vi "Snell_law.vi"(10 "Refr index":dbl=7.5, 11 "Angle in ext (deg)":dbl=7.5) -> (2 "Angle out int (deg)":dbl=7.5, 3 "Angle out int (rad)":dbl=7.5)   [LabVIEW 2012]
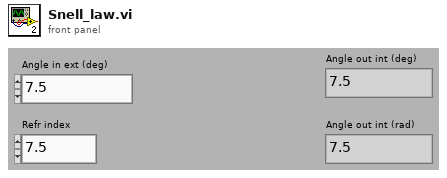
[diagram p1: front panel]
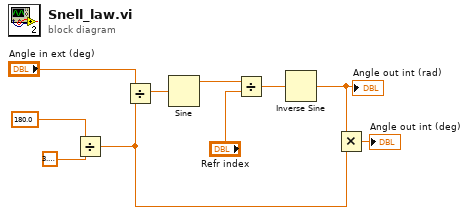
[diagram p0: block diagram]
diagram:
  n1 = Divide(x=sgl 180.0, y=3.141592653589793) -> (x/y=w1:dbl)
  n2 = Divide(x="Angle in ext (deg)", y=w1) -> (x/y=w7:dbl)
  n3 = Sine(x=w7) -> (sin(x)=w6:dbl)
  n4 = Divide(x=w6, y="Refr index") -> (x/y=w4:dbl)
  n5 = Inverse Sine(1:w4) -> (0:w3:dbl)
  "Angle out int (rad)" <- w3
  n6 = Multiply(x=w3, y=w1) -> (x*y=→"Angle out int (deg)":dbl)
